vi "serialreadfpga.vi"(2 "error in":errorcluster caption="error out", 7 "Timeout (ms)":i32=100, 9 "FPGA VI Reference In":refnum<k20>) -> (0 "Port5":string, 1 "Port8":string, 4 "FPGA VI Reference Out":refnum<k20>, 5 "Port6":string, 6 "Port1":string, 10 "Port2":string, 11 "Port4":string, 12 "Port7":string, 14 "Port3":string, 15 "error out":errorcluster)   [LabVIEW 2010]
uses:
  <vilib>/rvi/interface/nirviMethod/nirviMethod.xnode
  C:/Users/HAGAR-IV/Desktop/Zeugs/markus/version feb 2012/test/Auslesenkopiekopie2.vi
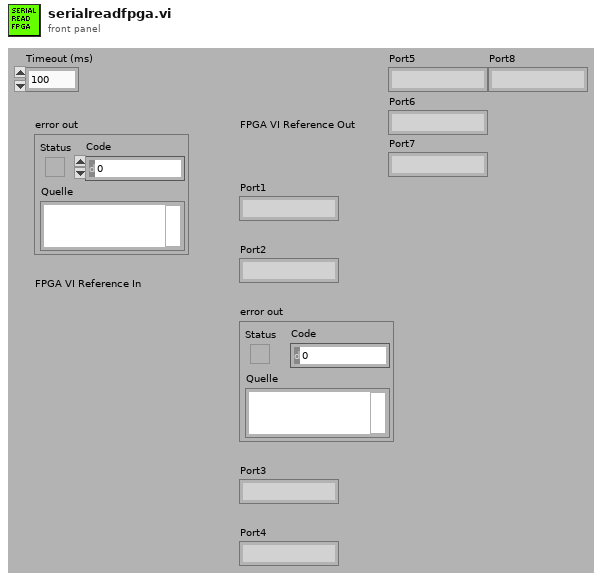
[diagram p1: front panel]
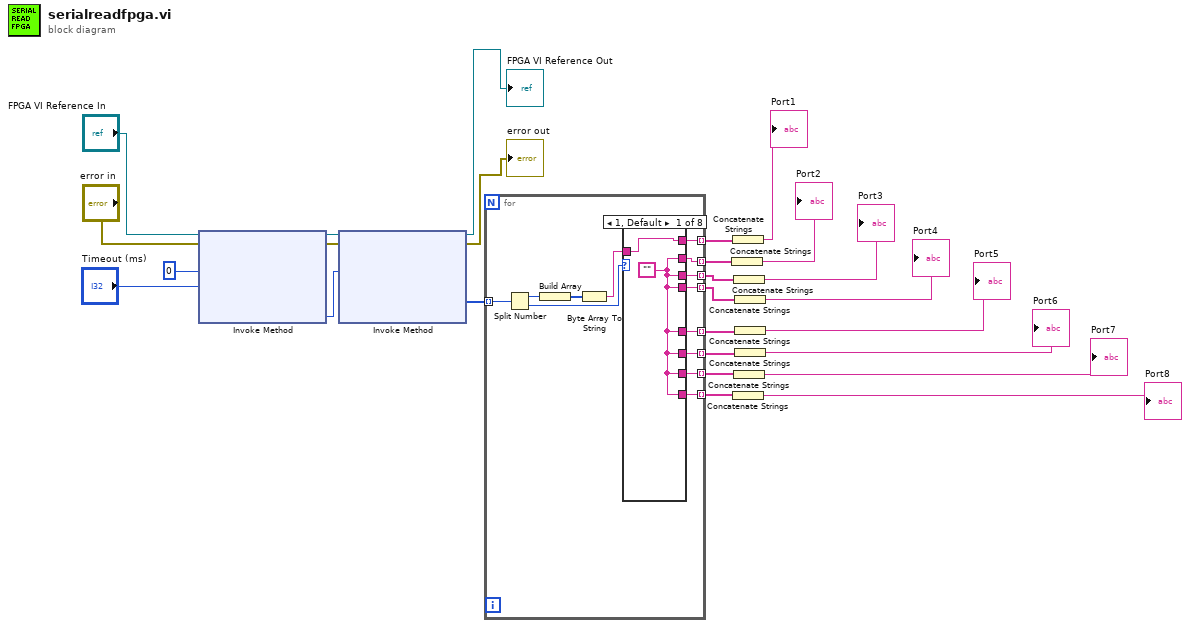
[diagram p0: block diagram]
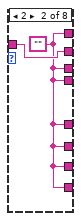
[diagram p2: hidden frame]
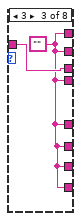
[diagram p3: hidden frame]
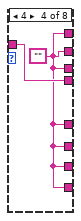
[diagram p4: hidden frame]
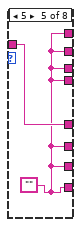
[diagram p5: hidden frame]
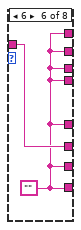
[diagram p6: hidden frame]
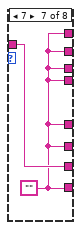
[diagram p7: hidden frame]
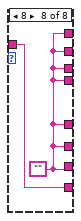
[diagram p8: hidden frame]
diagram:
  n1 = xnode "Invoke Method"("FPGA VI Reference In"="FPGA VI Reference In", "error in"="error in", "Number of Elements"=u32 0, "Timeout (ms)"="Timeout (ms)") -> ("FPGA VI Reference Out"=w11:refnum<k20>, "error out"=w12:errorcluster, "Elements Remaining"=w10:u32)  [unwired: 1 out]
  n2 = xnode "Invoke Method"("FPGA VI Reference In"=w11, "error in"=w12, "Number of Elements"=w10) -> ("FPGA VI Reference Out"=→"FPGA VI Reference Out":refnum<k20>, "error out"=→"error out":errorcluster, "Data"=w13:u16[])  [unwired: 2 out]
  n3 = for {
    tunnel: w13 -> [w39] mode=indexing
    tunnel: [w34] -> w21 mode=indexing
    tunnel: [w33] -> w22 mode=indexing
    tunnel: [w32] -> w20 mode=indexing
    tunnel: [w31] -> w19 mode=indexing
    tunnel: [w30] -> w8 mode=indexing
    tunnel: [w29] -> w7 mode=indexing
    tunnel: [w28] -> w6 mode=indexing
    tunnel: [w27] -> w5 mode=indexing
    n4 = Split Number(x=w39) -> (hi(x)=w38:u8, lo(x)=w36:u8)
    n5 = Build Array(w38) -> (w37:u8[])
    n6 = Byte Array To String(unsigned byte array=w37) -> (string=w35:string)
    n7 = case shown="1, Default" w36 {
      tunnel: w35 -> [w41 w43 w45 w47 w49 w51 w53 w55]
      tunnel: [w41 w42 w44 w46 w48 w50 w52 w54] -> w31
      tunnel: [w40 w42 w45 w46 w48 w50 w52 w54] -> w34
      tunnel: [w40 w42 w44 w47 w48 w50 w52 w54] -> w33
      tunnel: [w40 w43 w44 w46 w48 w50 w52 w54] -> w32
      tunnel: [w40 w42 w44 w46 w49 w50 w52 w54] -> w30
      tunnel: [w40 w42 w44 w46 w48 w51 w52 w54] -> w29
      tunnel: [w40 w42 w44 w46 w48 w50 w53 w54] -> w28
      tunnel: [w40 w42 w44 w46 w48 w50 w52 w55] -> w27
      frame 1, Default {
        w40 = ""
      }
      frame 2 {
        w42 = ""
      }
      frame 3 {
        w44 = ""
      }
      frame 4 {
        w46 = ""
      }
      frame 5 {
        w48 = ""
      }
      frame 6 {
        w50 = ""
      }
      frame 7 {
        w52 = ""
      }
      frame 8 {
        w54 = ""
      }
    }
  }
  n8 = Concatenate Strings(w20) -> (→"Port2":string)
  n9 = Concatenate Strings(w19) -> (→"Port1":string)
  n10 = Concatenate Strings(w5) -> (→"Port8":string)
  n11 = Concatenate Strings(w21) -> (→"Port3":string)
  n12 = Concatenate Strings(w6) -> (→"Port7":string)
  n13 = Concatenate Strings(w22) -> (→"Port4":string)
  n14 = Concatenate Strings(w8) -> (→"Port5":string)
  n15 = Concatenate Strings(w7) -> (→"Port6":string)
